vi "Fit Listbox to Pane.vi"(8 "error in (no error)":errorcluster, 10 "Owning Pane":refnum<vi>, 11 "Multicolumn Listbox":refnum<vi>) -> (0 "error out":errorcluster, 3 "Multicolumn Listbox":refnum<vi>)   [LabVIEW 2016]
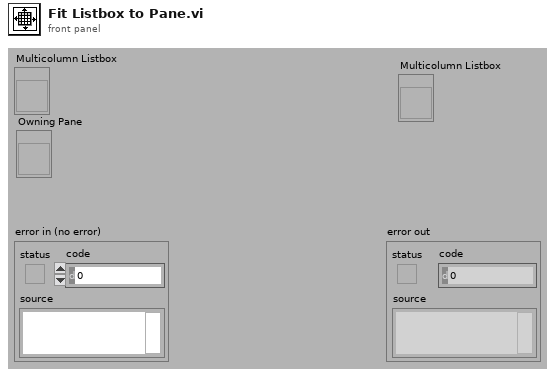
[diagram p1: front panel]
types:
  T1 = typedef "LVPositionTypeDef.ctl" = cluster{"Left":i32, "Top":i32}
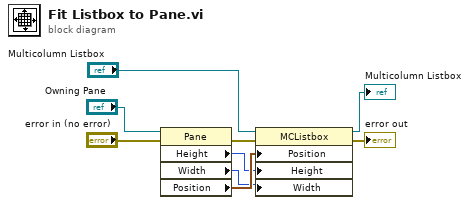
[diagram p0: block diagram]
diagram:
  n1 = property class="Pane"(reference="Owning Pane", error in="error in (no error)") -> (error out=w9:errorcluster, "Height"=w6:u32, "Width"=w5:u32, "Position"=w7:T1)  [unwired: 1 out]
  n2 = property class="MCListbox"(reference="Multicolumn Listbox", error in=w9, "Position"=w7, "Height"=w6, "Width"=w5) -> (reference out=→"Multicolumn Listbox":refnum<vi>, error out=→"error out":errorcluster)
